vi "salLabVIEWInterfaceMain.vi"() -> (0 "error out":errorcluster)   [LabVIEW 2013]
uses:
  PolymorphicStructure/PolymorphicStructure.lvclass
  PolymorphicStructure/PolymorphicStructure.lvclass/PolymorphicStructure.ctl
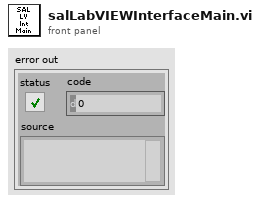
[diagram p1: front panel]
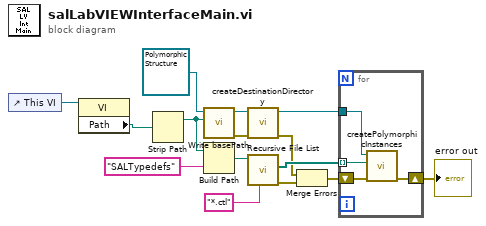
[diagram p0: block diagram]
diagram:
  n1 = control-ref of="This VI"() -> (w14:refnum<vi>)
  n2 = property class="VI"(reference=w14) -> ("Path"=w15:path)  [unwired: 1 in, 2 out]
  n3 = Strip Path(path=w15) -> (stripped path=w7:path)  [unwired: 1 out]
  n4 = call "Write basePath.vi"("basePath"=w7, "PolymorphicStructure in"=refnum<class "PolymorphicStructure.lvclass"> refnum) -> ("error out"=w11:errorcluster, "PolymorphicStructure out"=w12:refnum<class "PolymorphicStructure.lvclass">)  [unwired: 8 in]
  n5 = Build Path(base path=w7, name or relative path="SALTypedefs") -> (appended path=w6:path)
  n6 = call "createDestinationDirectory.vi"("error in (no error)"=w11, "PolymorphicStructure in"=w12) -> ("error out"=w3:errorcluster, "PolymorphicStructure out"=w9:refnum<class "PolymorphicStructure.lvclass">)  [unwired: 7 in, 1 out]
  n7 = call <vilib>:"Recursive File List.vi"("pattern"="*.ctl", "Folder Path"=w6) -> ("error out"=w2:errorcluster, "All Files in Dir"=w4:path[])  [unwired: 5 in, 3 out]
  n8 = Merge Errors(w3, w2) -> (w1:errorcluster)
  n9 = for {
    tunnel: w9 -> [w19]
    tunnel: w4 -> [w16] mode=indexing
    shift-right: [w17] -> w8
    shift-left: w1 -> [w18]
    n10 = call "createPolymorphicInstances.vi"("error in (no error)"=w18, "salTypdefPath"=w16, "PolymorphicStructure in"=w19) -> ("error out"=w17:errorcluster)  [unwired: 7 in, 1 out]
  }
  "error out" <- w8
